vi "read field (No Objects).vi"(8 "error in (no error)":errorcluster, 11 "Varian Magnet In":T2={"Fluke VISA resource name"="GPIB0::2::INSTR", "DAQ Physical Channel"="Dev1/ao0", "DAQ Task - Set"="", "DAQ Task - Read"="", "Control Voltage"=enum."40V", "extrapolated"={"x locations"=[], "coefficients"=[]}, "last 5 field numbers"=[], "Fluke Multimeter"={"function (0:volts DC)"=0, "range (0:auto)"=0, "rate (0:slow)"=0, "trigger mode (0:internal)"=0, "Autorange"=FALSE}} {"extrapolated"."x locations" format="%.4g"; "extrapolated"."coefficients" format="%.4g"; "Fluke Multimeter"."function (0:volts DC)" items=["volts DC", "volts AC", "2-wire k.ohms", "4-wire k.ohms", "mA DC", "mA AC"]; "Fluke Multimeter"."range (0:auto)" items=["autorange", "200mV, 200 ohms", "2V, 2 kohms", "20V, 20 kohms", "200V, 200 kohms", "1000Vdc, 700 Vac, 2 Mohms", "20 Mohms"]; "Fluke Multimeter"."rate (0:slow)" items=["slow", "medium", "fast"]; "Fluke Multimeter"."trigger mode (0:internal)" items=["internal - continuous trigger", "external - rear panel trigger with delay", "external - bus trigger with delay", "external - rear panel trigger", "external - bus trigger"]}) -> (0 "error out":errorcluster, 2 "Field":dbl[unit], 3 "Varian Magnet Out":T2={"Fluke VISA resource name"="GPIB0::2::INSTR", "DAQ Physical Channel"="Dev1/ao0", "DAQ Task - Set"="", "DAQ Task - Read"="", "Control Voltage"=enum."40V", "extrapolated"={"x locations"=[], "coefficients"=[]}, "last 5 field numbers"=[], "Fluke Multimeter"={"function (0:volts DC)"=0, "range (0:auto)"=0, "rate (0:slow)"=0, "trigger mode (0:internal)"=0, "Autorange"=FALSE}} {"extrapolated"."x locations" format="%.4g"; "extrapolated"."coefficients" format="%.4g"; "Fluke Multimeter"."function (0:volts DC)" items=["volts DC", "volts AC", "2-wire k.ohms", "4-wire k.ohms", "mA DC", "mA AC"]; "Fluke Multimeter"."range (0:auto)" items=["autorange", "200mV, 200 ohms", "2V, 2 kohms", "20V, 20 kohms", "200V, 200 kohms", "1000Vdc, 700 Vac, 2 Mohms", "20 Mohms"]; "Fluke Multimeter"."rate (0:slow)" items=["slow", "medium", "fast"]; "Fluke Multimeter"."trigger mode (0:internal)" items=["internal - continuous trigger", "external - rear panel trigger with delay", "external - bus trigger with delay", "external - rear panel trigger", "external - bus trigger"]})   [LabVIEW 2012]
doc: "Reads the current field."
uses:
  <vilib>/gmath/interp.llb/in_piecewise interp poly control.ctl
  Varian Constants (No Objects).vi
  <vilib>/gmath/NI_Gmath.lvlib
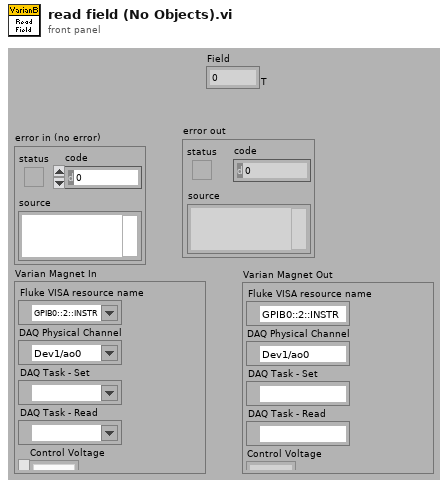
[diagram p1: front panel]
types:
  T1 = typedef "NI_Gmath.lvlib/in_piecewise interp poly control.ctl" = cluster{"x locations":dbl[], "coefficients":dbl[][]}
  T2 = cluster{"Fluke VISA resource name":refnum<visa-resource-name>, "DAQ Physical Channel":tag, "DAQ Task - Set":refnum<k21>, "DAQ Task - Read":refnum<k21>, "Control Voltage":enum16{"Please Select a Value", "30V", "40V"}, "extrapolated":T1, "last 5 field numbers":dbl[], "Fluke Multimeter":cluster{"function (0:volts DC)":u16, "range (0:auto)":u16, "rate (0:slow)":u16, "trigger mode (0:internal)":u16, "Autorange":bool}}
  T3 = cluster{"function (0:volts DC)":u16, "range (0:auto)":u16, "rate (0:slow)":u16, "trigger mode (0:internal)":u16, "Autorange":bool}
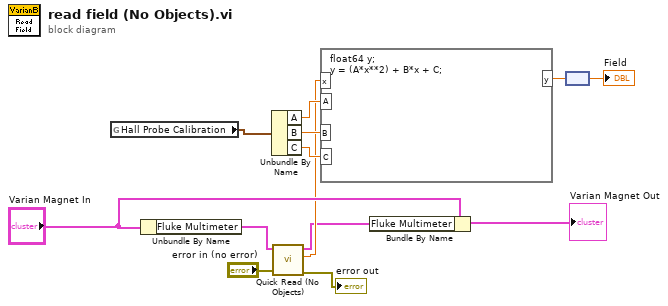
[diagram p0: block diagram]
diagram:
  n1 = global read "Varian Constants (No Objects).vi" "Hall Probe Calibration"() -> (w1:cluster{"A":dbl, "B":dbl, "C":dbl})
  n2 = Unbundle By Name("Varian Magnet In") -> ("Fluke Multimeter"=w4:T3)
  n3 = Unbundle By Name(w1) -> ("A"=w11:dbl, "B"=w10:dbl, "C"=w9:dbl)
  n4 = call "Quick Read (No Objects).vi"("error in (no error)"="error in (no error)", "Fluke Multimeter In"=w4) -> ("error out"=→"error out":errorcluster, "measurement"=w5:dbl, "Fluke Multimeter Out"=w2:T3)  [unwired: 6 in, 1 out]
  n5 = formula code="float64 y;\ny = (A*x**2) + B*x + C;"("x"=w5, "A"=w11, "B"=w10, "C"=w9) -> ("y"=w13:dbl)
  n6 = Bundle By Name(cluster="Varian Magnet In", "Fluke Multimeter"=w2) -> (→"Varian Magnet Out":T2)
  n7 = node(w13) -> (→"Field":dbl[unit])
